vi "CalculateFFT_v2.vi"(0 "Signals":waveform(dbl), 2 "Restart Averaging":bool, 5 "Spectrum Averaging Parameters":T2={"averaging mode"=1, "weighting mode"=0, "number of averages"=2} {"averaging mode" items=["No averaging", "Vector averaging", "RMS averaging", "Peak hold"]; "weighting mode" items=["Linear", "Exponential"]}, 7 "error in (no error)":errorcluster) -> (8 "FFT - (Peak)":cluster{"f0":dbl, "df":dbl, "magnitude":dbl[]}, 9 "averaging done":bool, 10 "Phase":cluster{"f0":dbl, "df":dbl, "phase":dbl[]}, 11 "error out":errorcluster)   [LabVIEW 2022 SP3]
uses:
  <vilib>/express/express analysis/Spectral/Block/exnSpectralBlock spectral measurements peak WFM.vi
panel:
  in  "View":T1={"dB On (F)"=TRUE, "unwrap phase (F)"=FALSE, "convert to degree (F)"=TRUE}
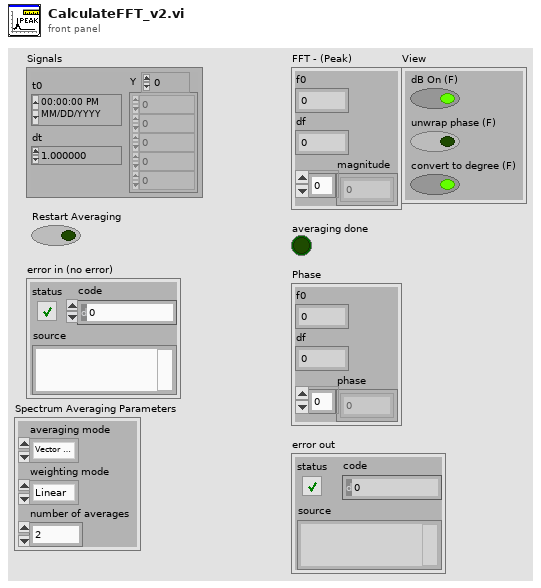
[diagram p1: front panel]
types:
  T1 = cluster{"dB On (F)":bool, "unwrap phase (F)":bool, "convert to degree (F)":bool}
  T2 = cluster{"averaging mode":u16, "weighting mode":u16, "number of averages":u32}
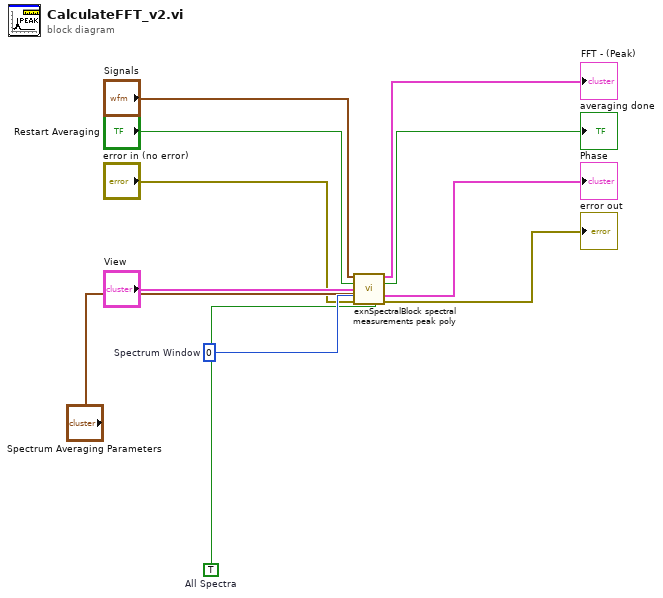
[diagram p0: block diagram]
diagram:
  w7 = TRUE  # All Spectra
  w9 = u16 0  # Spectrum Window
  n1 = call-poly <vilib>:"exnSpectralBlock spectral measurements peak poly.vi"("Signals"="Signals", "Restart Averaging"="Restart Averaging", "View"="View", "Spectrum Window"=w9, "error in (no error)"="error in (no error)", "Spectrum Averaging Parameters"="Spectrum Averaging Parameters", "All Spectra"=w7) -> ("Measurement Output"=→"FFT - (Peak)":cluster{"f0":dbl, "df":dbl, "magnitude":dbl[]}, "averaging done"=→"averaging done":bool, "Phase"=→"Phase":cluster{"f0":dbl, "df":dbl, "phase":dbl[]}, "error out"=→"error out":errorcluster)  [unwired: 5 in]
